vi "ENPH354_LabMG.vi"() -> ()   [LabVIEW 2020]
uses:
  <vilib>/MakerHub/LINX/Public/Peripherals/Digital/Digital Write 1 Chan.vi
  e283e988-d27c-4abd-8789-38d60b772bf2.vi
  <vilib>/MakerHub/LINX/Public/Peripherals/Analog/Analog Read 1 Chan.vi
  <vilib>/Analysis/baseanly.llb/Mean (DBL).vi
  <vilib>/MakerHub/LINX/Public/Peripherals/Digital/Digital Write N Chans.vi
  <vilib>/MakerHub/LINX/Public/Peripherals/Analog/Analog Read N Chans.vi
  <vilib>/MakerHub/LINX/Private/Local IO/LinxDigitalWrite.vi
  <vilib>/MakerHub/LINX/Public/Utilities/Check Channel.vi
  <vilib>/MakerHub/LINX/Private/Local IO/LinxAnalogRead.vi
  <vilib>/MakerHub/LINX/Public/Utilities/Open Serial.vi
  <vilib>/MakerHub/LINX/Private/Utilties/Generate Error.vi
  <vilib>/MakerHub/LINX/LMH-LINX.lvlib
  <vilib>/Analysis/NI_AALBase.lvlib
panel:
  out "LED On":bool
  in  "Final Angle [deg]":dbl
  in  "Initial Angle [deg]":dbl
  in  "Step Size [deg]":dbl
  out "error out":errorcluster
  in  "stop":bool
  out "Short Circuit Current vs Incident Angle":cluster{"X":dbl[], "Y":dbl[]}[](graph)
  out "Real Time Mean":dbl
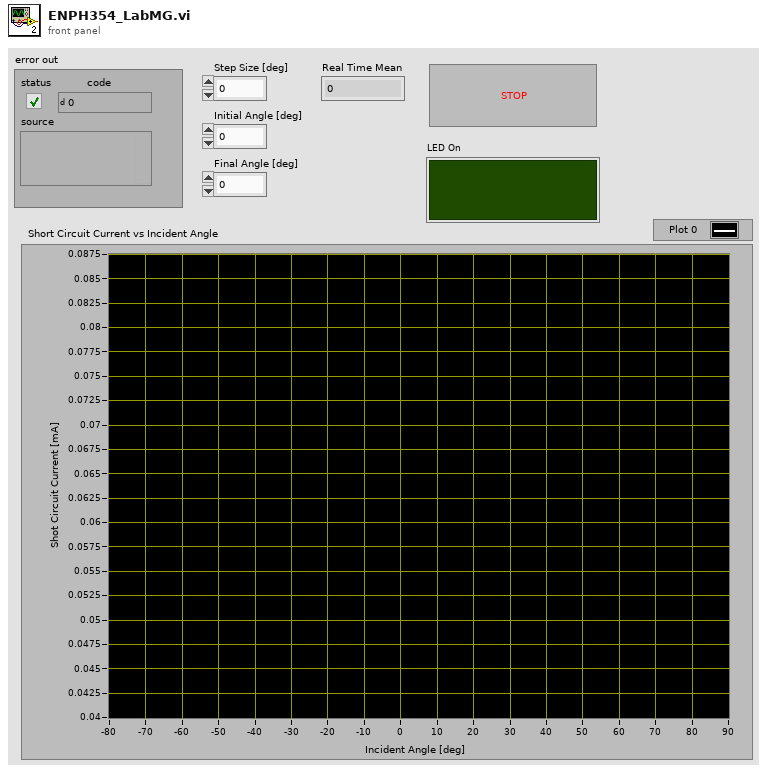
[diagram p1: front panel]
types:
  T1 = typedef "LMH-LINX.lvlib/LINX Ref.ctl" = cluster{"IO":T2, "Interface":T3, "LINX Device Config":T4}
  T2 = typedef "LMH-LINX.lvlib/Platform.ctl" = enum16{"Remote", "Local"}
  T3 = typedef "LMH-LINX.lvlib/Interface.ctl" = enum16{"Serial", "TCP"}
  T4 = typedef "LMH-LINX.lvlib/Device.lvlib/LINX Device Config.ctl" = cluster{"Interface":T3, "COM Port":refnum<visa-resource-name>, "TCP Configuration":T5, "Device Family":u8, "Device ID":u8, "Device Name":string, "TCP Ref":refnum<k5>, "Channels":T6}
  T5 = typedef "LMH-LINX.lvlib/Device.lvlib/TCP Config.ctl" = cluster{"IP Address":string, "Port":u16}
  T6 = typedef "LMH-LINX.lvlib/Channels.ctl" = cluster{"DI":u8[], "DO":u8[], "AI":u8[], "AO":u8[], "PWM":u8[], "QE":u8[], "UART":u8[], "I2C 2":u8[], "SPI":u8[], "CAN":u8[], "Servo":u8[], "AI Ref (V)":dbl, "AI Resolution (Bits)":u8, "AO Ref (V)":dbl, "AO Resolution (Bits)":u8}
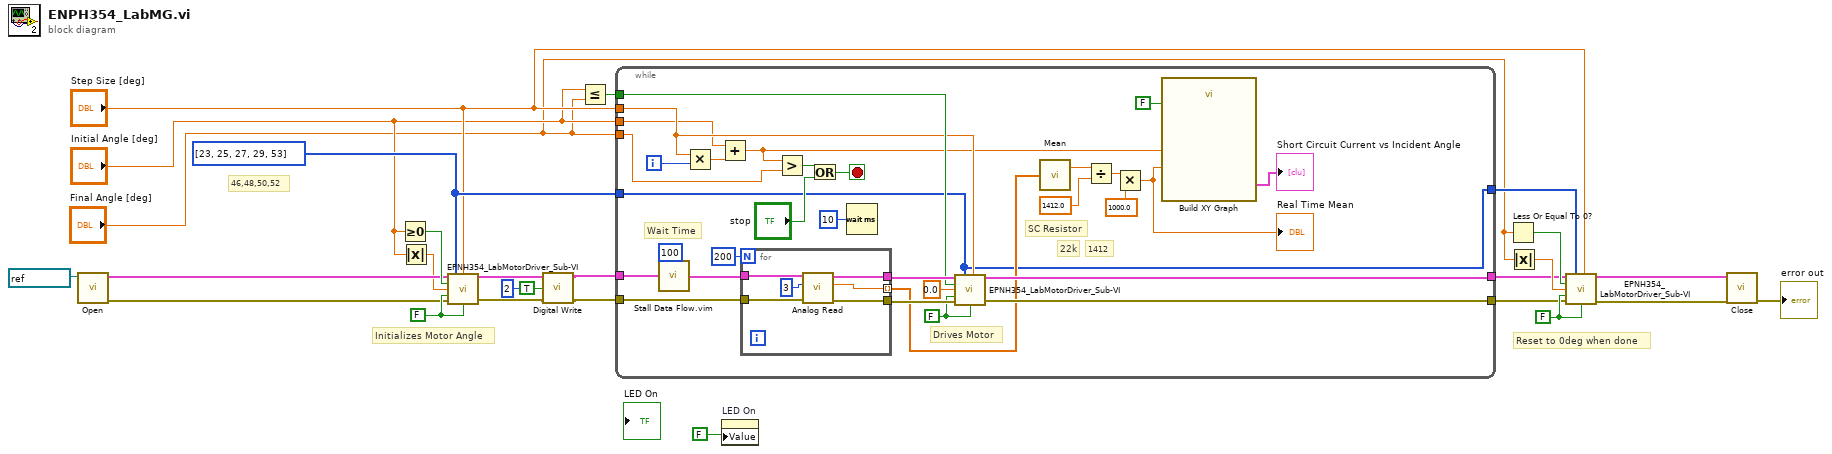
[diagram p0: block diagram]
diagram:
  w21 = FALSE ("stop in")
  w17 = i32[] [23, 25, 27, 29, 53] ("Array")
  w24 = FALSE ("Run Continuous in")
  # "Reset to 0deg when done"
  # "46,48,50,52"
  # "Initializes Motor Angle"
  n1 = call-poly <vilib>:"Open.vi"("Serial Port"=refnum<visa-resource-name> "COM4") -> ("Error Out"=w18:errorcluster, "LINX Resource"=w19:T1)  [unwired: 8 in, 1 out]
  n2 = Greater Or Equal To 0?(x="Initial Angle [deg]") -> (x >= 0?=w25:bool)
  n3 = Absolute Value(x="Initial Angle [deg]") -> (abs(x)=w10:dbl)
  n4 = call "EPNH354_LabMotorDriver_Sub-VI.vi"("LINX Resource in"=w19, "Array"=w17, "Step Size in"="Step Size [deg]", "Run Clockwise in"=w25, "Rotation Range in"=w10, "Run Continuous in"=w24, "error in (no error)"=w18, "stop in"=w24) -> ("LINX Resource out"=w4:T1, "error out"=w3:errorcluster)  [unwired: 6 in]
  n5 = call-poly <vilib>:"Digital Write.vi"("Error In"=w3, "Output Value"=TRUE, "DO Channel"=u8 2 ("PWM Channel"), "LINX Resource"=w4) -> ("Error Out"=w5:errorcluster, "LINX Resource"=w6:T1)  [unwired: 6 in]
  n6 = Less Or Equal?(x="Initial Angle [deg]", y="Final Angle [deg]") -> (x <= y?=w20:bool)
  n7 = while {
    tunnel: w6 -> [w50]
    tunnel: w5 -> [w49]
    tunnel: [w56] -> w16
    tunnel: [w55] -> w15
    tunnel: "Initial Angle [deg]" -> [w39]
    tunnel: "Step Size [deg]" -> [w40]
    tunnel: "Final Angle [deg]" -> [w31]
    tunnel: w17 -> [w33]
    tunnel: w20 -> [w42]
    tunnel: [w33] -> w11
    i -> [w38]
    stop <- w35 stop-if-true
    w48 = FALSE ("stop in")
    # "1412"
    # "22k"
    # "Drives Motor"
    # "SC Resistor"
    # "Wait Time"
    n8 = call "Stall Data Flow.vim"("value in"=w50, "milliseconds to wait"=u32 100) -> ("value out"=w52:T1)  [unwired: 1 out]
    n9 = Multiply(x=w40, y=w38) -> (x*y=w41:dbl)
    n10 = Add(x=w39, y=w41) -> (x+y=w32:dbl)
    n11 = for {
      N: 200 -> [_]
      tunnel: w52 -> [w64]
      tunnel: w49 -> [w63]
      tunnel: [w61] -> w34 mode=indexing
      tunnel: [w60] -> w54
      tunnel: [w59] -> w53
      n12 = call-poly <vilib>:"Analog Read.vi"("Error In"=w63, "Analog Channel"=u8 3, "LINX Resource"=w64) -> ("Error Out"=w59:errorcluster, "Voltage"=w61:dbl, "LINX Resource"=w60:T1)  [unwired: 5 in, 1 out]
    }
    n13 = Greater?(x=w32, y=w31) -> (0:w37:bool)
    n14 = Or(x=w37, y="stop") -> (x .or. y?=w35:bool)
    n15 = Wait (ms)(milliseconds to wait=u32 10) -> ()  [unwired: 1 out]
    n16 = call "EPNH354_LabMotorDriver_Sub-VI.vi"("LINX Resource in"=w54, "Array"=w33, "Step Size in"=w40, "Run Clockwise in"=w42, "Rotation Range in"=0.0, "Run Continuous in"=w48, "error in (no error)"=w53, "stop in"=w48) -> ("LINX Resource out"=w56:T1, "error out"=w55:errorcluster)  [unwired: 6 in]
    n17 = call-poly <vilib>:"Mean.vi"("X"=w34) -> ("mean"=w46:dbl)  [unwired: 1 out]
    n18 = Divide(x=w46, y=1412.0) -> (x/y=w30:dbl)
    n19 = Multiply(x=w30, y=1000.0) -> (x*y=w28:dbl)
    "Real Time Mean" <- w28
    n20 = call "Build XY Graph"("Reset"=FALSE, "Y Input"=w28, "X Input"=w32) -> ("XY Graph"=→"Short Circuit Current vs Incident Angle":cluster{"X":dbl[], "Y":dbl[]}[])  [unwired: 7 in, 1 out]
  }
  n21 = property on="LED On" class="Bool (strict)"("Value"=FALSE ("Indicator")) -> ()  [unwired: 2 in, 2 out]
  n22 = Less Or Equal To 0?(x="Final Angle [deg]") -> (x <= 0?=w23:bool)
  n23 = Absolute Value(x="Final Angle [deg]") -> (abs(x)=w22:dbl)
  n24 = call "EPNH354_LabMotorDriver_Sub-VI.vi"("LINX Resource in"=w16, "Array"=w11, "Step Size in"="Step Size [deg]", "Run Clockwise in"=w23, "Rotation Range in"=w22, "Run Continuous in"=w21, "error in (no error)"=w15, "stop in"=w21) -> ("LINX Resource out"=w14:T1, "error out"=w13:errorcluster)  [unwired: 6 in]
  n25 = call <vilib>:"Close.vi"("Error In"=w13, "LINX Resource"=w14) -> ("Error Out"=→"error out":errorcluster)  [unwired: 9 in]
